vi "Get TOF LUT.vi"() -> (2 "Info":cluster{i32, i32}, 3 "LUT Out":dbl[](array[numeric]))   [LabVIEW 2025]
panel:
  in  "TOF LUT":dbl[](array[numeric])=[1.22, 1.31, 1.38, 1.4, 1.67]
  in  "Outputs":cluster{"Min Setpoint":i32, "Max Setpoint":i32}
  out "Max Hood Setpoint":i32
  out "Min Hood Setpoint":i32
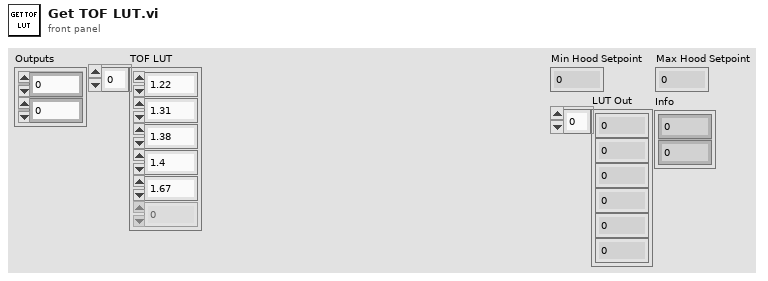
[diagram p1: front panel]
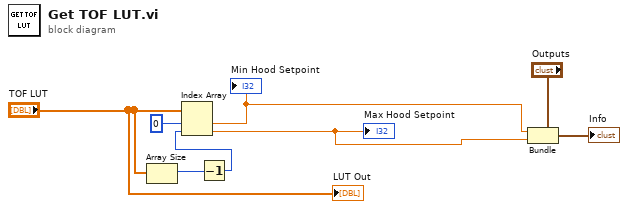
[diagram p0: block diagram]
diagram:
  n1 = Array Size(array="TOF LUT") -> (size(s)=w7:i32)
  n2 = Decrement(x=w7) -> (x-1=w5:i32)
  n3 = Index Array(array="TOF LUT", index #1=0 ("index"), index #2=w5) -> (element #1=w6:dbl, element #2=w4:dbl)
  "Min Hood Setpoint" <- w6
  "Max Hood Setpoint" <- w4
  n4 = Bundle(cluster="Outputs", "Min Setpoint"=w6, "Max Setpoint"=w4) -> (→"Info":cluster{"Min Setpoint":i32, "Max Setpoint":i32})
  "LUT Out" <- "TOF LUT"
